vi "7-4_max30102HR.vi"() -> ()   [LabVIEW 2014]
doc: "Use this template to build a producer/consumer design pattern. Use this template when you need to execute a process, such as data analysis, when a data source, such as a triggered acquisition, produces data at an uneven rate and you need to execute the process when the data becomes available.\n------------------------------------\nAuther: Koji Ohashi\nCopyright (c) 2020 Japan LabVIEW Users Group, Volunteer members.\nThis VI is released under the MIT License.\nhttp://opensource.org/licenses/mit-license.php\n------------------------------------"
uses:
  <vilib>/Instr/_visa.llb/VISA Configure Serial Port (Instr).vi
  <vilib>/measure/NI_MAPro.lvlib
  <vilib>/measure/matone.llb/Extract Single Tone Information 1 Chan.vi
panel:
  out "Heart rate":dbl
  out "Waveform Graph":waveform(dbl)(graph)
  in  "Read Count":u32=1000
  in  "Termination Character":u8=10 format="%.0x"
  in  "VISA resource name":refnum<visa-resource-name>="COM1"
  in  "Serial Settings":T1={"baud rate"=9600, "data bits"=8, "parity"=enum."None", "stop bits"=10, "flow control"=0} {"flow control" items=["None"=0, "XON/XOFF"=1, "RTS/CTS"=2, "DTR/DSR"=4]; "stop bits" items=["1.0"=10, "1.5"=15, "2.0"=20]; "data bits" min=5 max=8 step=1; "baud rate" items=["75"=75, "110"=110, "134"=134, "150"=150, "300"=300, "600"=600, "1200"=1200, "1800"=1800, "2400"=2400, "4800"=4800, "7200"=7200, "9600"=9600, "14400"=14400, "19200"=19200, "28800"=28800, "38400"=38400, "56000"=56000, "57600"=57600, "115200"=115200, "128000"=128000, "230400"=230400]}
  in  "End Read on Termination Character?":bool=TRUE
  in  "stop":bool
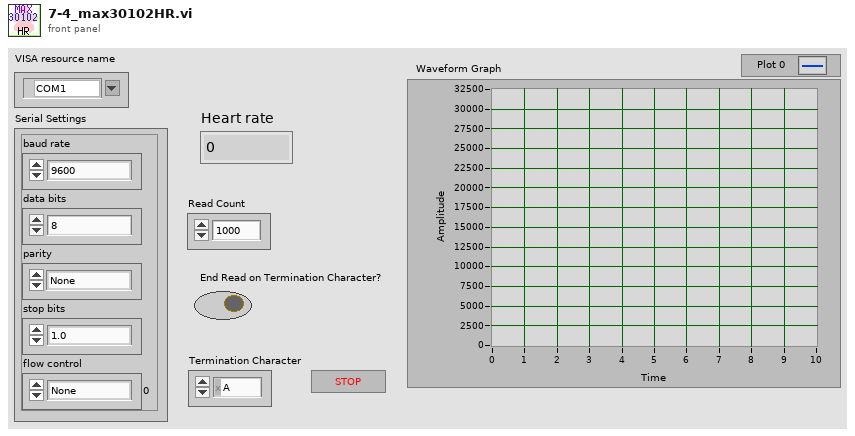
[diagram p1: front panel]
types:
  T1 = cluster{"baud rate":u32, "data bits":u16, "parity":enum16{"None", "Odd", "Even", "Mark", "Space"}, "stop bits":u16, "flow control":u16}
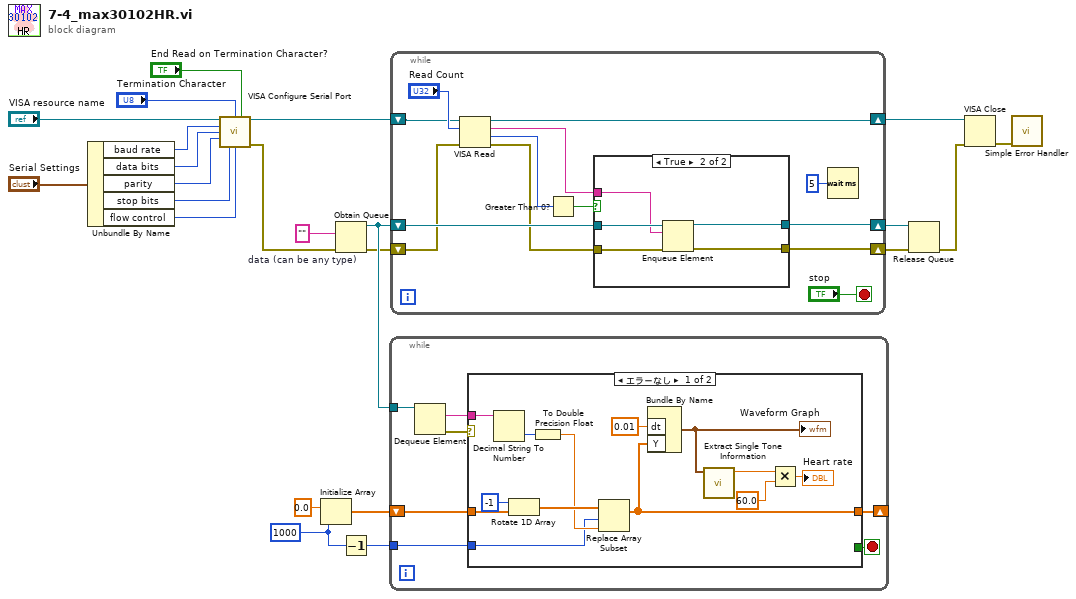
[diagram p0: block diagram]
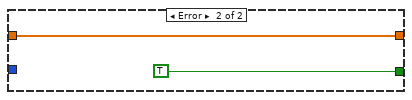
[diagram p2: hidden frame]
diagram:
  w2 = 1000 ("dimension size")
  w19 = ""  # data (can be any type)
  n1 = Unbundle By Name("Serial Settings") -> ("baud rate"=w14:u32, "data bits"=w15:u16, "parity"=w16:enum16{"None", "Odd", "Even", "Mark", "Space"}, "stop bits"=w17:u16, "flow control"=w11:u16)
  n2 = call-poly "VISA Configure Serial Port"("VISA resource name"="VISA resource name", "termination char\n(0xA = '\\n' = LF)"="Termination Character", "Enable Termination\nChar (T)"="End Read on Termination Character?", "baud rate (9600)"=w14, "data bits (8)"=w15, "parity (0:none)"=w16, "stop bits (10: 1 bit)"=w17, "flow control (0:none)"=w11) -> ("VISA resource name out"=w9:refnum<visa-resource-name>, "error out"=w6:errorcluster)  [unwired: 2 in, 4 out]
  n3 = Initialize Array "Initialize Array"(0.0 ("element"), w2) -> (w3:dbl[])
  n4 = Obtain Queue(element data type=w19, error in (no error)=w6) -> (queue out=w23:refnum<queue>, error out=w22:errorcluster)  [unwired: 3 in, 1 out]
  n5 = Decrement(x=w2) -> (x-1=w1:i32)
  n6 = while {
    tunnel: w23 -> [w30]
    shift-right: [w25] -> _
    shift-left: w3 -> [w26]
    tunnel: w1 -> [w24]
    stop <- w27 stop-if-true
    n7 = Dequeue Element(queue=w30) -> (element=w28:string, error out=w29:errorcluster)  [unwired: 2 in, 2 out]
    n8 = case shown="エラーなし" w29 {
      tunnel: w28 -> [w43 _]
      tunnel: [_ TRUE] -> w27
      tunnel: w26 -> [w42 w44]
      tunnel: [w36 w44] -> w25
      tunnel: w24 -> [w31 _]
      frame No Error {
        n9 = Decimal String To Number(string=w43) -> (number=w39:i32)  [unwired: 2 in, 1 out]
        n10 = Rotate 1D Array(1:w42, 2:-1 ("n")) -> (0:w40:dbl[])
        n11 = To Double Precision Float(number=w39) -> (double precision float=w38:dbl)
        n12 = Replace Array Subset "Replace Array Subset"(array=w40, new element=w38, index=w31) -> (w36:dbl[])
        n13 = Bundle By Name("dt"=0.01, "Y"=w36) -> (w35:waveform(dbl))  [unwired: 1 in]
        "Waveform Graph" <- w35
        n14 = call-poly <vilib>:"Extract Single Tone Information.vi"("time signal in"=w35) -> ("detected frequency"=w33:dbl)  [unwired: 5 in, 5 out]
        n15 = Multiply(x=w33, y=60.0) -> (x*y=→"Heart rate":dbl)
      }
      frame Error {
      }
    }
  }
  n16 = while {
    shift-right: [w55] -> w20
    shift-left: w22 -> [w48]
    shift-right: [w56] -> w21
    shift-left: w23 -> [w57]
    shift-right: [w52] -> w7
    shift-left: w9 -> [w46]
    stop <- "stop" stop-if-true
    n17 = VISA Read(VISA resource name=w46, byte count="Read Count", error in (no error)=w48) -> (VISA resource name out=w52:refnum<visa-resource-name>, read buffer=w49:string, return count=w51:u32, error out=w47:errorcluster)
    n18 = Greater Than 0?(x=w51) -> (x > 0?=w50:bool)
    n19 = case shown="TRUE" w50 {
      tunnel: w57 -> [w60 w65]
      tunnel: [w60 w64] -> w56
      tunnel: w47 -> [w59 w63]
      tunnel: [w59 w62] -> w55
      tunnel: w49 -> [_ w61]
      frame False {
      }
      frame True {
        n20 = Enqueue Element(queue=w65, element=w61, error in (no error)=w63) -> (queue out=w64:refnum<queue>, error out=w62:errorcluster)  [unwired: 1 in, 1 out]
      }
    }
    n21 = Wait (ms)(milliseconds to wait=u32 5) -> ()  [unwired: 1 out]
  }
  n22 = Release Queue(queue=w21, error in (no error)=w20) -> (error out=w5:errorcluster)  [unwired: 1 in, 2 out]
  n23 = VISA Close(VISA resource name=w7, error in (no error)=w5) -> (error out=w8:errorcluster)
  n24 = call <vilib>:"Simple Error Handler.vi"("error in (no error)"=w8) -> ()  [unwired: 1 in, 8 out]
